vi "CRC16 USB.vi"(5 "data":string) -> (2 "crc":string)   [LabVIEW 2021]
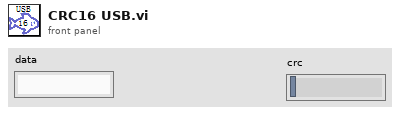
[diagram p1: front panel]
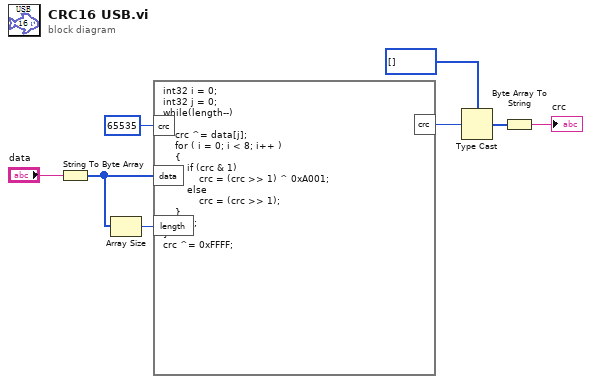
[diagram p0: block diagram]
diagram:
  n1 = String To Byte Array(string="data") -> (unsigned byte array=w7:u8[])
  n2 = Array Size(array=w7) -> (size(s)=w6:i32)
  n3 = formula code="int32 i = 0;\nint32 j = 0;\nwhile(length--)\n{\n    crc ^= data[j]; \n    for ( i = 0; i < 8; i++ )\n    {\n        if (crc & 1)\n            crc = (crc >> 1) ^ 0xA001;\n        else\n            crc = (crc >> 1);\n    }\n    j++;\n}\ncrc ^= 0xFFFF;"("data"=w7, "length"=w6, "crc"=u16 65535) -> ("crc"=w3:u16)
  n4 = Type Cast(type=u8[] [] ("unsigned byte array"), x=w3) -> (*(type *) &x=w1:u8[])
  n5 = Byte Array To String(unsigned byte array=w1) -> (string=→"crc":string)
